vi "Set Temperature.vi"(8 "error in (no error)":errorcluster, 9 "Internal?":bool, 10 "Setpoint":dbl, 11 "Lauda Settings In":T1) -> (0 "error out":errorcluster, 1 "Connection Error":bool, 3 "Lauda Settings Out":T1)   [LabVIEW 2018, in "Lauda TCU.lvlib"]
uses:
  Lauda TCU.lvlib
  Lauda Settings.ctl
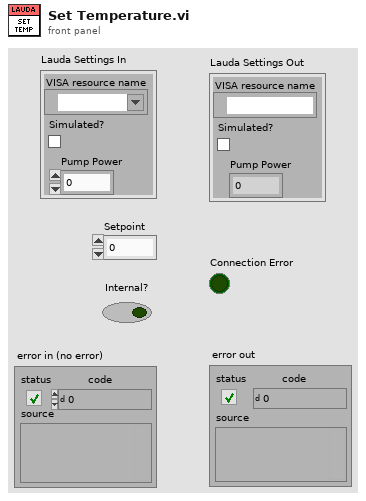
[diagram p1: front panel]
types:
  T1 = typedef "Lauda TCU.lvlib/Lauda Settings.ctl" = cluster{"VISA resource name":refnum<visa-resource-name>, "Simulated?":bool, "Pump Power":i32}
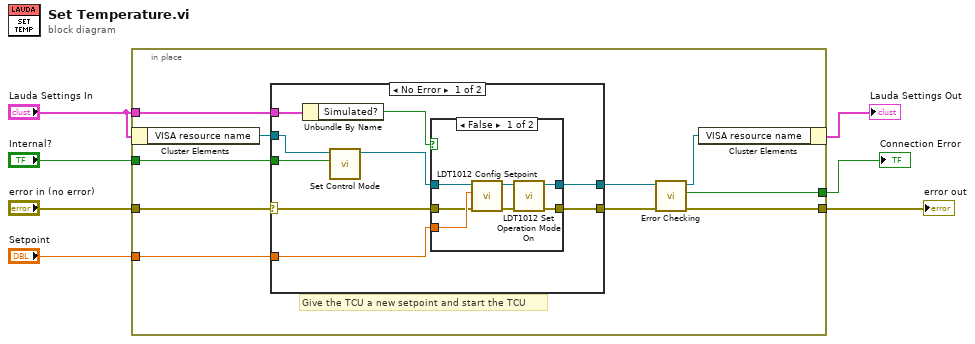
[diagram p0: block diagram]
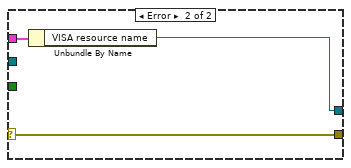
[diagram p3: hidden frame]
diagram:
  n1 = in-place {
    in-place-border: "error in (no error)" -> [w17]
    in-place-border: [w14] -> w6
    in-place-border: "Lauda Settings In" -> [w13]
    in-place-border: [w12] -> w5
    in-place-border: "Internal?" -> [w11]
    in-place-border: "Setpoint" -> [w8]
    # "Give the TCU a new setpoint and start the TCU"
    n2 = in-place-cluster #1("Lauda Settings In") -> ("VISA resource name"=w10:refnum<visa-resource-name>)
    n3 = case shown="No Error" w17 {
      selector: w17 -> [w26 w38]
      tunnel: w13 -> [w22 w37]
      tunnel: [w25 w38] -> w15
      tunnel: [w24 w36] -> w16
      tunnel: w11 -> [w21 _]
      tunnel: w10 -> [w19 _]
      tunnel: w8 -> [w18 _]
      frame No Error {
        n4 = Unbundle By Name(w22) -> ("Simulated?"=w23:bool)
        n5 = call "Set Control Mode.vi"("Internal Control"=w21, "VISA session"=w19) -> ("dup VISA session"=w20:refnum<visa-resource-name>)  [unwired: 8 in, 1 out]
        n6 = case shown="False" w23 {
          tunnel: w26 -> [w31 w35]
          tunnel: [w27 w35] -> w25
          tunnel: [w28 w34] -> w24
          tunnel: w20 -> [w33 w34]
          tunnel: w18 -> [w32 _]
          frame False {
            n7 = call "LDT1012 Config Setpoint.vi"("error in (no error)"=w31, "Setpoint (20.00 °C: Default)"=w32, "VISA session"=w33) -> ("error out"=w30:errorcluster, "dup VISA session"=w29:refnum<visa-resource-name>)  [unwired: 7 in]
            n8 = call "LDT1012 Set Operation Mode On.vi"("error in (no error)"=w30, "VISA session"=w29) -> ("error out"=w27:errorcluster, "dup VISA session"=w28:refnum<visa-resource-name>)  [unwired: 8 in]
          }
          frame True {
          }
        }
      }
      frame Error {
        n9 = Unbundle By Name(w37) -> ("VISA resource name"=w36:refnum<visa-resource-name>)
      }
    }
    n10 = call "Error Checking.vi"("error in (no error)"=w15, "VISA resource name"=w16) -> ("error out"=w14:errorcluster, "Connection Error"=w12:bool, "VISA resource name"=w9:refnum<visa-resource-name>)  [unwired: 7 in]
    n11 = in-place-cluster #1("VISA resource name"=w9) -> (→"Lauda Settings Out":T1)
  }
  "error out" <- w6
  "Connection Error" <- w5
